vi "Test S-Matrix API.vi"() -> ()   [LabVIEW 2016]
doc: "S-Matrix API Tester."
uses:
  S-Matrix.lvlib
  <vilib>/Utility/error.llb/DialogType.ctl
  Initialize Parameter.ctl
  <instrlib>/niSwitch/niSwitch.llb/niSwitch Topologies.ctl
panel:
  in  "VISA resource name":refnum<visa-resource-name>
  in  "topology name":T1="2737/2-Wire 4x64 Matrix" caption="Topology Name"
  in  "REQ Disconnect Channel":bool
  in  "Second Connection":cluster{"channel 3":string, "channel 4":string}={"channel 3"="r1", "channel 4"="c1"}
  in  "First Connection":cluster{"channel 1":string, "channel 2":string}={"channel 1"="r0", "channel 2"="c0"}
  in  "REQ Making Connection":bool
  in  "REQ Close Ref":bool
  in  "relay action":i32(ring)=21 caption="Relay Action" items=["Open Relay"=20, "Close Relay"=21]
  in  "relay name":string="k0" caption="Relay Name"
  in  "REQ Single Relay":bool
  in  "DAQ Type":enum16{"Hardware", "Simulation"}(ring)
  out "Connect?":bool
  in  "REQ Initialize Hardware":bool
  in  "Show Diagram on Init":bool
  in  "Show Block Diagram":bool
  in  "Stop Module":bool
  in  "Start Module":bool
  in  "Hide Module Panel":bool
  in  "Show Module Panel":bool
  out "Status":string
  out "Module Running?":bool
  # "This VI tests the API for the Module."
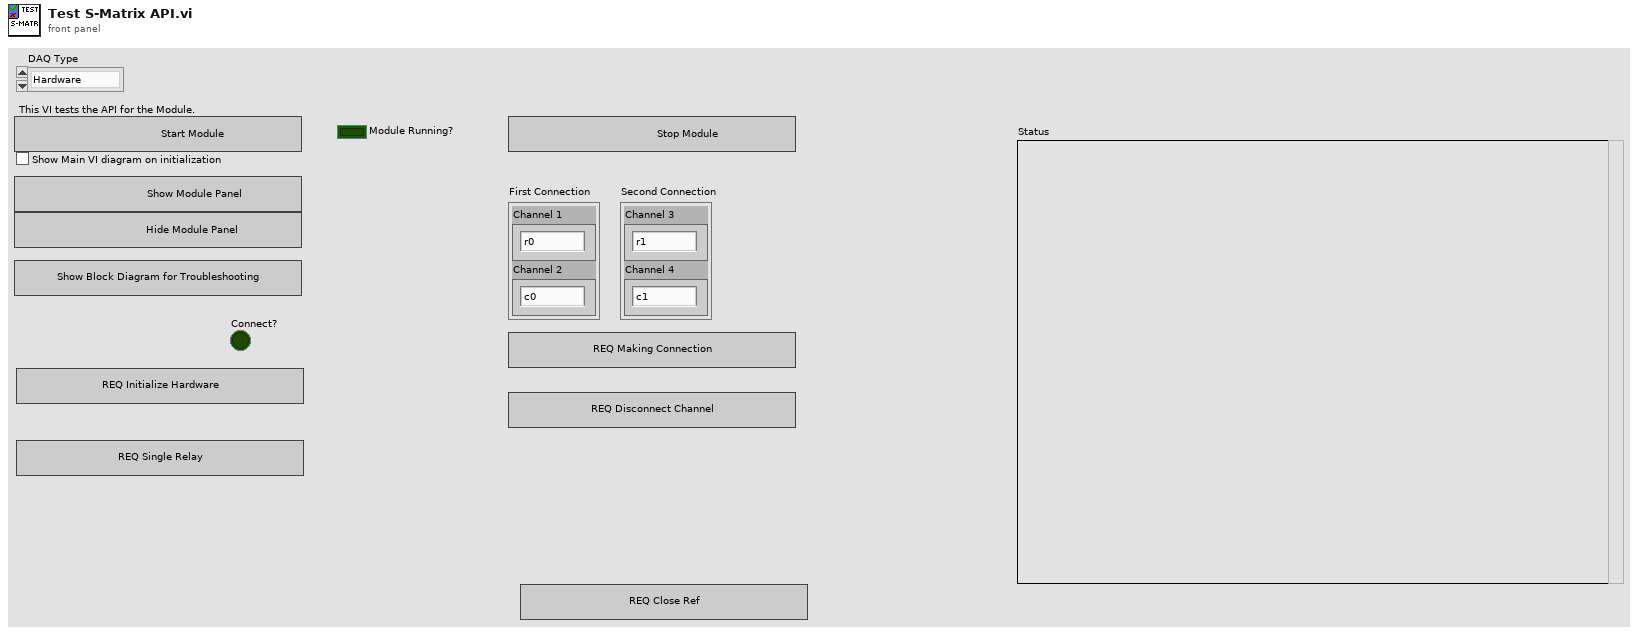
[diagram p1: front panel]
types:
  T1 = typedef "niSwitch Topologies.ctl" = string
  T2 = typedef "S-Matrix.lvlib/Broadcast Events--cluster.ctl" = cluster{"Module Did Init":refnum<user-event>, "Status Updated":refnum<user-event>, "Error Reported":refnum<user-event>, "Module Did Stop":refnum<user-event>, "Update Module Execution Status":refnum<user-event>}
  T3 = typedef "S-Matrix.lvlib/Initialize Parameter.ctl" = cluster{"Ref":variant, "topology name":string}
  T4 = typedef "DialogType.ctl" = u16
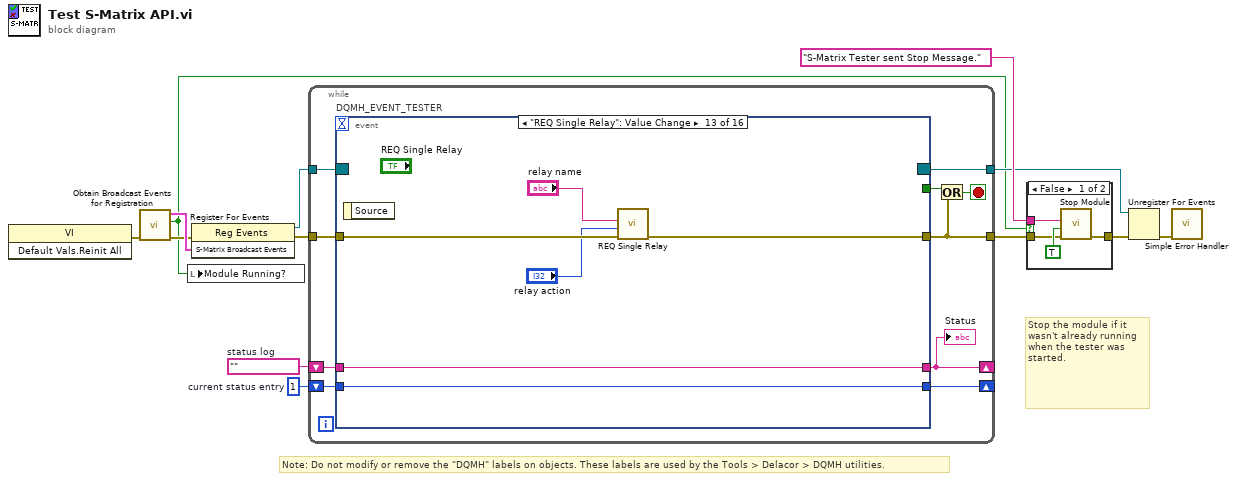
[diagram p0: block diagram]
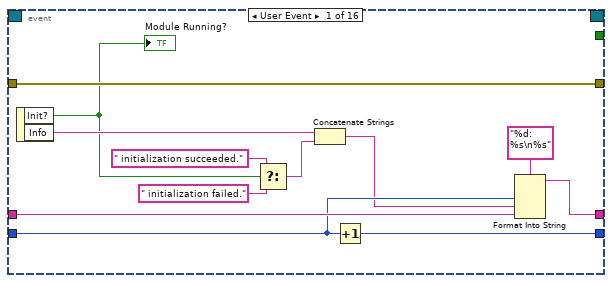
[diagram p3: hidden frame]
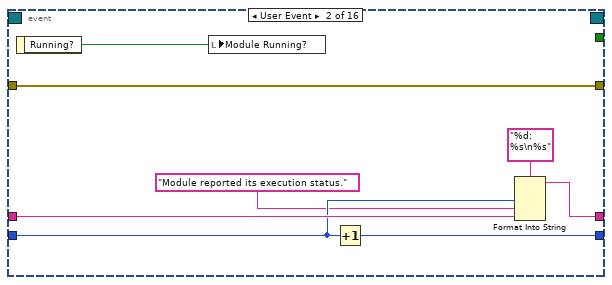
[diagram p4: hidden frame]
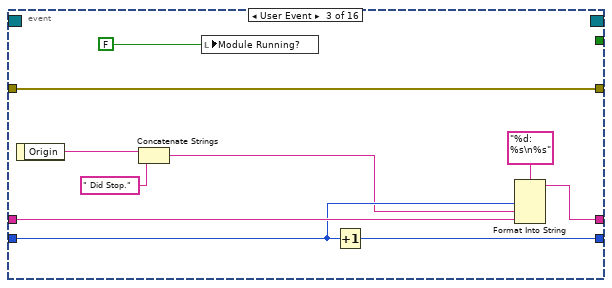
[diagram p5: hidden frame]
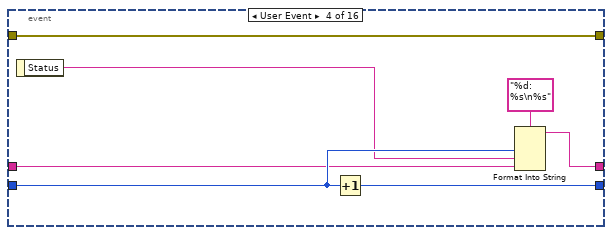
[diagram p6: hidden frame]
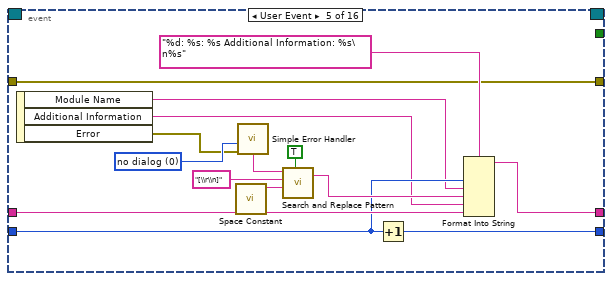
[diagram p7: hidden frame]
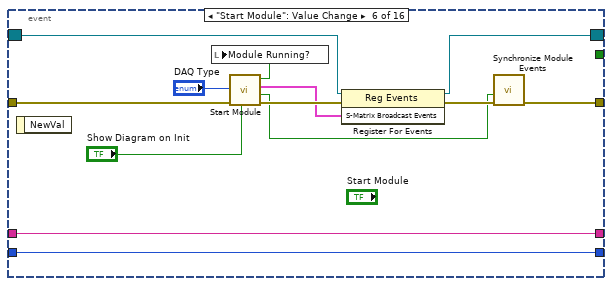
[diagram p8: hidden frame]
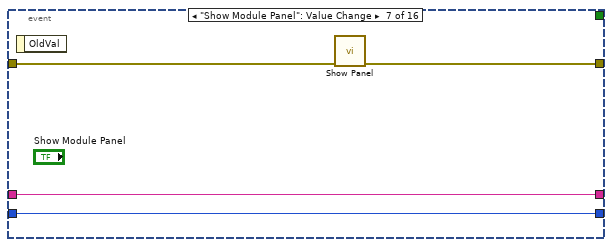
[diagram p9: hidden frame]
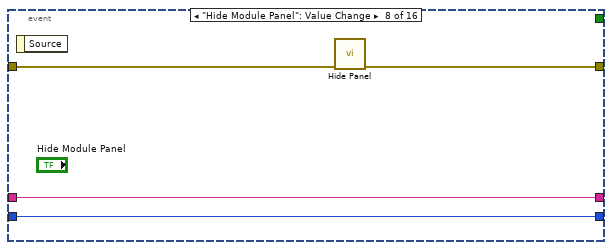
[diagram p10: hidden frame]
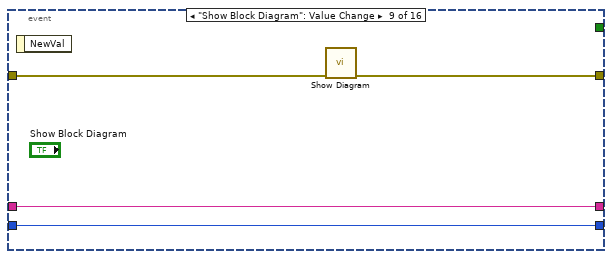
[diagram p11: hidden frame]
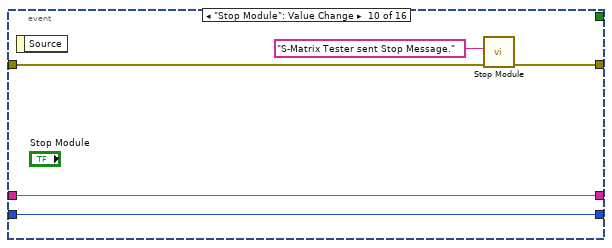
[diagram p12: hidden frame]
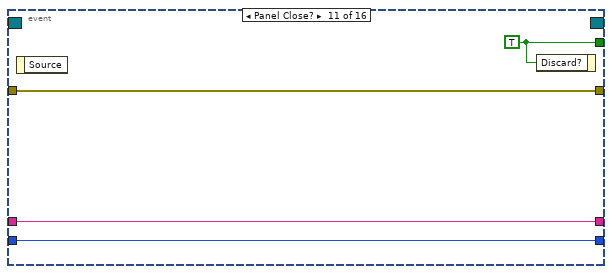
[diagram p13: hidden frame]
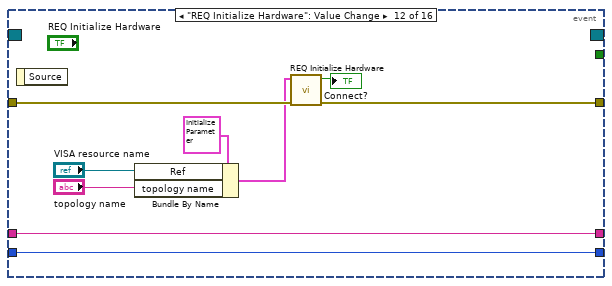
[diagram p14: hidden frame]
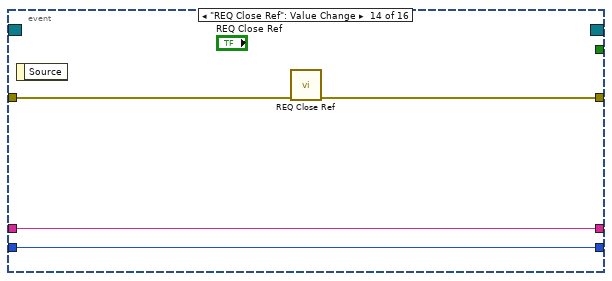
[diagram p15: hidden frame]
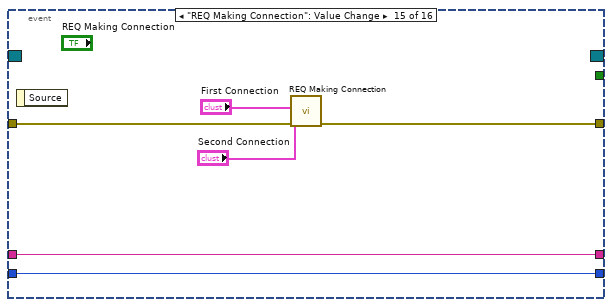
[diagram p16: hidden frame]
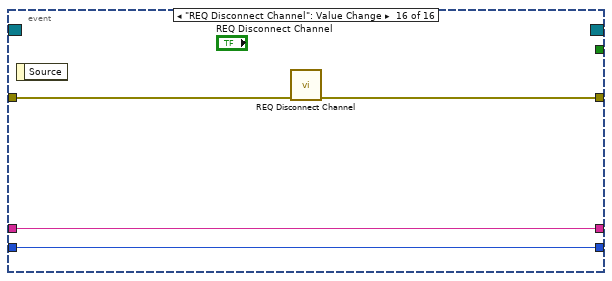
[diagram p17: hidden frame]
diagram:
  w10 = 1  # current status entry
  w11 = ""  # status log
  # "Stop the module if it wasn't already running when the tester was started."
  # "Note: Do not modify or remove the \"DQMH\" labels on objects. These labels are used by the Tools > Delacor > DQMH utilities."
  n1 = invoke class="VI" method="Default Vals.Reinit All"() -> (error out=w5:errorcluster)  [unwired: 3 in, 2 out]
  n2 = call "Obtain Broadcast Events for Registration.vi"("error in"=w5) -> ("error out"=w4:errorcluster, "Already running?"=w3:bool, "S-Matrix Broadcast Events"=w8:T2)  [unwired: 8 in]
  n3 = local write "Module Running?"(w3) -> ()
  n4 = register-events(error in=w4, w8) -> (reference out=w7:refnum<event-registration>, error out=w9:errorcluster)  [unwired: 1 in]
  n5 = while {
    tunnel: w7 -> [w23]
    tunnel: [w14] -> w2
    shift-right: [w18] -> _
    shift-left: w11 -> [w20]
    shift-right: [w19] -> _
    shift-left: w10 -> [w21]
    tunnel: w9 -> [w16]
    tunnel: [w15] -> w6
    stop <- w17 stop-if-true
    n6 = event "DQMH_EVENT_TESTER" shown="[12] \"REQ Single Relay\": Value Change" {
      selector: w23 -> [_ _ _ _ _ w82 _ _ _ _ _ _ _ _ _ _]
      dyn-events: [_ _ _ _ _ w81 _ _ _ _ _ _ _ _ _ _] -> w15
      timeout: _ -> [_ _ _ _ _ _ _ _ _ _ _ _ _ _ _ _]
      tunnel: [_ _ _ _ _ _ _ _ _ _ w109 _ _ _ _ _] -> w22
      tunnel: [w35 w37 w44 w54 w64 w80 w92 w96 w97 w103 w106 w115 w121 w125 w131 w135] -> w14
      tunnel: w21 -> [w32 w41 w51 w57 w67 w85 w90 w94 w98 w104 w107 w116 w122 w126 w132 w136]
      tunnel: w20 -> [w33 w42 w52 w56 w68 w86 w91 w95 w99 w105 w108 w117 w123 w127 w133 w137]
      tunnel: [w30 w39 w49 w58 w66 w86 w91 w95 w99 w105 w108 w117 w123 w127 w133 w137] -> w18
      tunnel: [w31 w40 w50 w60 w65 w85 w90 w94 w98 w104 w107 w116 w122 w126 w132 w136] -> w19
      tunnel: w16 -> [w35 w37 w44 w54 w64 w79 w89 w93 w100 w101 w106 w118 w124 w128 w134 w138]
      event User Event {
        n7 = event-data() -> ("Init?"=w27:bool, "Info"=w29:string)  [unwired: 1 in]
        "Module Running?" <- w27
        n8 = Select(t=" initialization succeeded.", s=w27, f=" initialization failed.") -> (s? t:f=w24:string)
        n9 = Concatenate Strings(w29, w24) -> (w28:string)
        n10 = Increment(x=w32) -> (x+1=w31:i32)
        n11 = Format Into String(format string="%d: %s\n%s", w32, w28, w33) -> (resulting string=w30:string)  [unwired: 2 in, 1 out]
      }
      event User Event {
        n12 = event-data() -> ("Running?"=w36:bool)  [unwired: 1 in]
        n13 = local write "Module Running?"(w36) -> ()
        n14 = Increment(x=w41) -> (x+1=w40:i32)
        n15 = Format Into String(format string="%d: %s\n%s", w41, "Module reported its execution status.", w42) -> (resulting string=w39:string)  [unwired: 2 in, 1 out]
      }
      event User Event {
        n16 = event-data() -> ("Origin"=w48:string)  [unwired: 1 in]
        n17 = Concatenate Strings(w48, " Did Stop.") -> (w47:string)
        n18 = local write "Module Running?"(FALSE ("Module Did Init?")) -> ()
        n19 = Increment(x=w51) -> (x+1=w50:i32)
        n20 = Format Into String(format string="%d: %s\n%s", w51, w47, w52) -> (resulting string=w49:string)  [unwired: 2 in, 1 out]
      }
      event User Event {
        n21 = event-data() -> ("Status"=w55:string)  [unwired: 1 in]
        n22 = Increment(x=w57) -> (x+1=w60:i32)
        n23 = Format Into String(format string="%d: %s\n%s", w57, w55, w56) -> (resulting string=w58:string)  [unwired: 2 in, 1 out]
      }
      event User Event {
        w69 = T4 0 items=["no dialog", "OK message", "continue or stop message", "OK message + warnings", "continue/stop + warnings"] ("type of dialog (OK msg:1)")
        n24 = event-data() -> ("Module Name"=w63:string, "Additional Information"=w62:string, "Error"=w61:errorcluster)  [unwired: 1 in]
        n25 = call <vilib>:"Space Constant.vi"() -> ("String"=w73:string)
        n26 = call <vilib>:"Simple Error Handler.vi"("type of dialog (OK msg:1)"=w69, "error in (no error)"=w61) -> ("message"=w70:string)  [unwired: 3 in, 4 out]
        n27 = call <vilib>:"Search and Replace Pattern.vi"("string"=w70, "regular expression (\"\")"="[\\r\\n]" ("regular expression (\"\")"), "replace string (\"\")"=w73, "replace all? (F)"=TRUE ("replace all CR/LF with spaces")) -> ("result string"=w71:string)  [unwired: 1 in, 1 out]
        n28 = Increment(x=w67) -> (x+1=w65:i32)
        n29 = Format Into String(format string="%d: %s: %s Additional Information: %s\n%s", w67, w63, w71, w62, w68) -> (resulting string=w66:string)  [unwired: 2 in, 1 out]
      }
      event "Start Module": Value Change {
        n30 = event-data() -> ()  [unwired: 1 in, 1 out]
        n31 = call "Start Module.vi"("Show Main VI Diagram on Init (F)"="Show Diagram on Init", "error in"=w79, "DAQ Type"="DAQ Type") -> ("error out"=w87:errorcluster, "Wait for Event Sync?"=w84:bool, "S-Matrix Broadcast Events"=w83:T2, "Module Was Already Running?"=w78:bool)  [unwired: 5 in]
        n32 = local write "Module Running?"(w78) -> ()
        n33 = register-events(reference=w82, error in=w87, w83) -> (reference out=w81:refnum<event-registration>, error out=w88:errorcluster)
        n34 = call "Synchronize Module Events.vi"("error in"=w88, "Wait for Event Sync?"=w84) -> ("error out"=w80:errorcluster)  [unwired: 9 in]
      }
      event "Show Module Panel": Value Change {
        n35 = event-data() -> ()  [unwired: 1 in, 1 out]
        n36 = call "Show Panel.vi"("error in (no error)"=w89) -> ("error out"=w92:errorcluster)  [unwired: 10 in]
      }
      event "Hide Module Panel": Value Change {
        n37 = event-data() -> ()  [unwired: 1 in, 1 out]
        n38 = call "Hide Panel.vi"("error in (no error)"=w93) -> ("error out"=w96:errorcluster)  [unwired: 10 in]
      }
      event "Show Block Diagram": Value Change {
        n39 = event-data() -> ()  [unwired: 1 in, 1 out]
        n40 = call "Show Diagram.vi"("error in (no error)"=w100) -> ("error out"=w97:errorcluster)  [unwired: 10 in]
      }
      event "Stop Module": Value Change {
        n41 = event-data() -> ()  [unwired: 1 in, 1 out]
        n42 = call "Stop Module.vi"("error in"=w101, "Origin"="S-Matrix Tester sent Stop Message.") -> ("error out"=w103:errorcluster)  [unwired: 9 in]
      }
      event Panel Close? {
        w109 = TRUE ("Discard?")
        n43 = event-data() -> ()  [unwired: 1 in, 1 out]
        n44 = event-data("Discard?"=w109) -> ()  [unwired: 1 in, 1 out]
      }
      event "REQ Initialize Hardware": Value Change {
        n45 = event-data() -> ()  [unwired: 1 in, 1 out]
        n46 = Bundle By Name(cluster=T3 {"Ref"=variant, "topology name"="Configured Topology"} ("Initialize Parameter"), "Ref"="VISA resource name", "topology name"="topology name") -> (w110:T3)
        n47 = call "REQ Initialize Hardware.vi"("error in"=w118, "Initialize Parameter"=w110) -> ("error out"=w115:errorcluster, "Connect?"=→"Connect?":bool)  [unwired: 7 in, 1 out]
      }
      event "REQ Single Relay": Value Change {
        n48 = event-data() -> ()  [unwired: 1 in, 1 out]
        n49 = call "REQ Single Relay.vi"("error in"=w124, "relay action"="relay action", "relay name"="relay name") -> ("error out"=w121:errorcluster)  [unwired: 8 in]
      }
      event "REQ Close Ref": Value Change {
        n50 = event-data() -> ()  [unwired: 1 in, 1 out]
        n51 = call "REQ Close Ref.vi"("error in"=w128) -> ("error out"=w125:errorcluster)  [unwired: 10 in]
      }
      event "REQ Making Connection": Value Change {
        n52 = event-data() -> ()  [unwired: 1 in, 1 out]
        n53 = call "REQ Making Connection.vi"("error in"=w134, "Second Connection"="Second Connection", "First Connection"="First Connection") -> ("error out"=w131:errorcluster)  [unwired: 8 in]
      }
      event "REQ Disconnect Channel": Value Change {
        n54 = event-data() -> ()  [unwired: 1 in, 1 out]
        n55 = call "REQ Disconnect Channel.vi"("error in"=w138) -> ("error out"=w135:errorcluster)  [unwired: 10 in]
      }
    }
    "Status" <- w18
    n56 = Or(x=w22, y=w14) -> (x .or. y?=w17:bool)
  }
  n57 = case shown="False" w3 {
    tunnel: [w142 w143] -> w13
    tunnel: "S-Matrix Tester sent Stop Message." ("Origin") -> [w141 _]
    tunnel: w2 -> [w139 w143]
    frame False {
      n58 = call "Stop Module.vi"("error in"=w139, "Wait for Module to Stop? (F)"=TRUE ("Wait for Module to stop?"), "Origin"=w141) -> ("error out"=w142:errorcluster)  [unwired: 8 in]
    }
    frame True {
    }
  }
  n59 = Unregister For Events(event registration refnum=w6, error in=w13) -> (error out=w1:errorcluster)
  n60 = call <vilib>:"Simple Error Handler.vi"("error in (no error)"=w1) -> ()  [unwired: 4 in, 5 out]
